vi "to_json.vi"(8 "error in":errorcluster, 11 "endingTimestamp in":refnum<class "endingTimestamp.lvclass">) -> (0 "error out":errorcluster, 2 "json":string, 3 "endingTimestamp out":refnum<class "endingTimestamp.lvclass">, 4 "Not Default":bool)   [LabVIEW 2020, in "nominal types.lvlib" / "timestampManifest.lvlib" / "endingTimestamp.lvclass"]
uses:
  endingTimestamp.lvclass
  endingTimestamp.lvclass/endingTimestamp.ctl
  4a6799ba-c5e5-4c66-8feb-5e644ce3fb2d.vi
  <vilib>/JDP Science/JSONtext/Variant to JSON Text.vi
  <vilib>/JDP Science/JSONtext/LVClass Serializer/JSONtext LVClass Serializer.lvclass
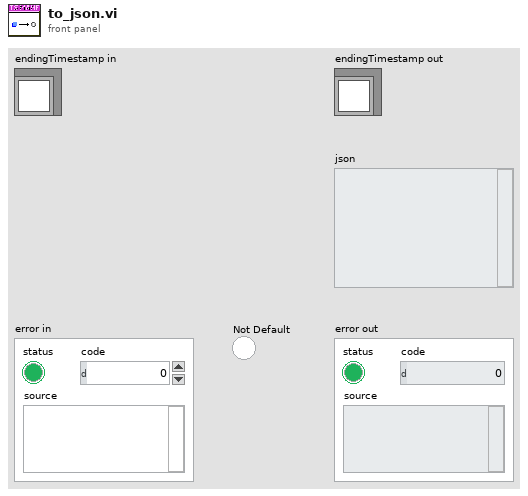
[diagram p1: front panel]
types:
  T1 = cluster{"type":string, "endingTimestamp":cluster{"seconds":i64, "nanos":i64, "picos":i64}}
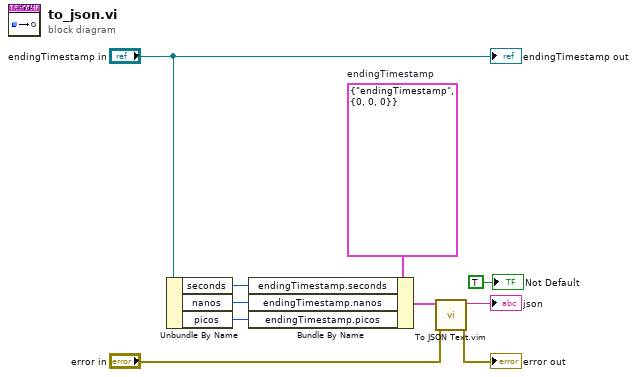
[diagram p0: block diagram]
diagram:
  w10 = T1 {"type"="endingTimestamp", "endingTimestamp"={"seconds"=0, "nanos"=0, "picos"=0}}  # endingTimestamp
  n1 = Unbundle By Name("endingTimestamp in") -> ("seconds"=w5:i64, "nanos"=w6:i64, "picos"=w7:i64)
  n2 = Bundle By Name(cluster=w10, "endingTimestamp.seconds"=w5, "endingTimestamp.nanos"=w6, "endingTimestamp.picos"=w7) -> (w9:T1)
  n3 = call "To JSON Text.vim"("error in (no error)"="error in", "Anything"=w9) -> ("error out"=→"error out":errorcluster, "<JSON>"=→"json":string)  [unwired: 8 in]
  "endingTimestamp out" <- "endingTimestamp in"
  "Not Default" <- TRUE ("Not Default")
